vi "Start Create.vi"(9 "Alias":string, 10 "Actor":refnum<class "Actor.lvclass">, 11 "TEMPLATE Actor in":refnum<class "TEMPLATE Actor.lvclass">) -> (0 "Error out":errorcluster, 3 "TEMPLATE Actor out":refnum<class "TEMPLATE Actor.lvclass">)   [LabVIEW 2020, in "_Template.lvlib" / "Templates.lvlib" / "TEMPLATE Actor.lvlib" / "TEMPLATE Actor.lvclass"]
uses:
  TEMPLATE Actor.lvclass
  jettl/jettl/Actor/Actor/Actor.lvclass
  TEMPLATE Actor.lvclass/TEMPLATE Actor.ctl
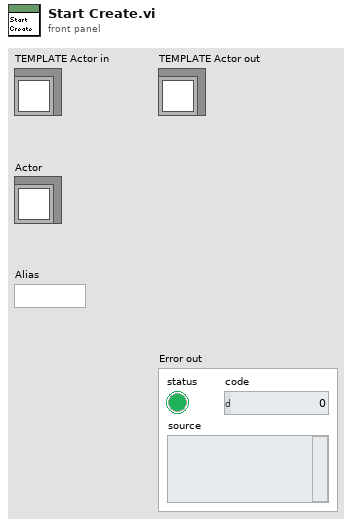
[diagram p1: front panel]
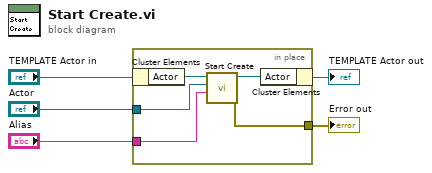
[diagram p0: block diagram]
diagram:
  n1 = in-place {
    in-place-border: "Alias" -> [w7]
    in-place-border: "Actor" -> [w8]
    in-place-border: [w6] -> w2
    n2 = in-place-cluster #1("TEMPLATE Actor in") -> ("Actor"=w10:refnum<class "Actor.lvclass">)
    n3 = call-dynamic "Start Create.vi"("Alias"=w7, "Actor"=w8, "Actor in"=w10) -> ("Error out"=w6:errorcluster, "Actor out"=w9:refnum<class "Actor.lvclass">)  [unwired: 7 in]
    n4 = in-place-cluster #1("Actor"=w9) -> (→"TEMPLATE Actor out":refnum<class "TEMPLATE Actor.lvclass">)
  }
  "Error out" <- w2
